vi "Finish.vi"   [LabVIEW 2018]
doc: "This VI is called just before exiting. It is expected to close I/O refnum, save collected data, etc."
uses:
  <vilib>/Rock Robotics/WPI/Utilities/WPI_GetSetVariantRefNum.vi
  <vilib>/Rock Robotics/WPI/Ultrasonic/WPI_SonarSRF04DigitalRefNum Registry Get.vi
  <vilib>/Rock Robotics/WPI/Ultrasonic/WPI_SonarSRF04DigitalClose.vi
types:
  T1 = typedef "WPI_JoystickDevRef.ctl" = cluster{"Device":T2}
  T2 = typedef "WPI_JoystickDeviceEnum.ctl" = enum16{"USB 0", "USB 1", "USB 2", "USB 3", "USB 4", "USB 5"}
  T3 = typedef "WPI_CompressorDevRef.ctl" = cluster{"DevStatus":errorcluster, "Pneumatics Control Module":u8}
  T4 = typedef "WPI_RobotDriveDevRef.ctl" = cluster{"DevStatus":errorcluster, "Motors[]":T5[], "Square Inputs":bool, "Max Output":dbl}
  T5 = typedef "WPI_MotorControlDeviceRef.ctl" = cluster{"DeviceStatus":errorcluster, "Type":T6, "PWM":cluster{"PWM Channel":T7, "DeadBand":T8}, "CAN":cluster{"Device Number":u8, "SetOutput VI Ref":variant, "GetOutput VI Ref":variant, "Enable VI Ref":variant, "Disable VI Ref":variant, "Data":variant}, "Invert":bool, "DIO PWM":cluster{"PWM \"Enable\" Channel":T7, "DIOChannel":T9, "PWM Rate":dbl}}
  T6 = typedef "WPI_MotorControlType.ctl" = enum16{"PWM", "CAN", "DIO PWM"}
  T7 = typedef "FPGA_DIOPWMChannel.ctl" = enum8{"PWM 0", "PWM 1", "PWM 2", "PWM 3", "PWM 4", "PWM 5", "PWM 6", "PWM 7", "PWM 8", "PWM 9", "PWM MXP 0", "PWM MXP 1", "PWM MXP 2", "PWM MXP 3", "PWM MXP 4", "PWM MXP 5", "PWM MXP 6", "PWM MXP 7", "PWM MXP 8", "PWM MXP 9", "Invalid"}
  T8 = typedef "WPI_PWMDeadband.ctl" = cluster{"Name":string, "maxPositivePwm":i32, "minPositivePwm":i32, "centerPwm":i32, "maxNegativePwm":i32, "minNegativePwm":i32, "angularRange":u16}
  T9 = typedef "FPGA_DIOChannel.ctl" = enum8{"DIO 0", "DIO 1", "DIO 2", "DIO 3", "DIO 4", "DIO 5", "DIO 6", "DIO 7", "DIO 8", "DIO 9", "DIO MXP 0", "DIO MXP 1", "DIO MXP 2", "DIO MXP 3", "DIO MXP 4", "DIO MXP 5", "DIO MXP 6", "DIO MXP 7", "DIO MXP 8", "DIO MXP 9", "DIO MXP 10", "DIO MXP 11", "DIO MXP 12", "DIO MXP 13", "DIO MXP 14", "DIO MXP 15", "SPI Port CS1", "SPI Port CS2", "SPI Port CS3", "SPI Port MISO", "SPI Port MOSI", "Invalid"}
  T10 = typedef "WPI_EncoderDevRef.ctl" = cluster{"DevStatus":errorcluster, "EncoderIndex":T11, "CounterIndex":T12, "DistancePerCount":dbl, "Decoding Type":T13}
  T11 = typedef "FPGA_EncoderIdx.ctl" = enum8{"Enc 0", "Enc 1", "Enc 2", "Enc 3", "Enc 4", "Enc 5", "Enc 6", "Enc 7", "Invalid"}
  T12 = typedef "FPGA_CounterCtrSystemIndex.ctl" = enum8{"Ctr 0", "Ctr 1", "Ctr 2", "Ctr 3", "Ctr 4", "Ctr 5", "Ctr 6", "Ctr 7", "Invalid"}
  T13 = typedef "WPI_EncoderType.ctl" = enum16{"1x", "2x", "4x"}
  T14 = typedef "WPI_SwitchDevRef.ctl" = cluster{"DevStatus":errorcluster, "DIO Channel":T9, "CntIndex":T12, "Normally Closed":bool}
  T15 = typedef "WPI_UltrasonicDeviceRef.ctl" = cluster{"DevStatus":errorcluster, "Ping Channel":T9, "Echo Channel":T9, "CntIndex":T12}
  T16 = typedef "WPI_CameraDevRef.ctl" = cluster{"Camera Address":string, "CameraStatus":errorcluster}
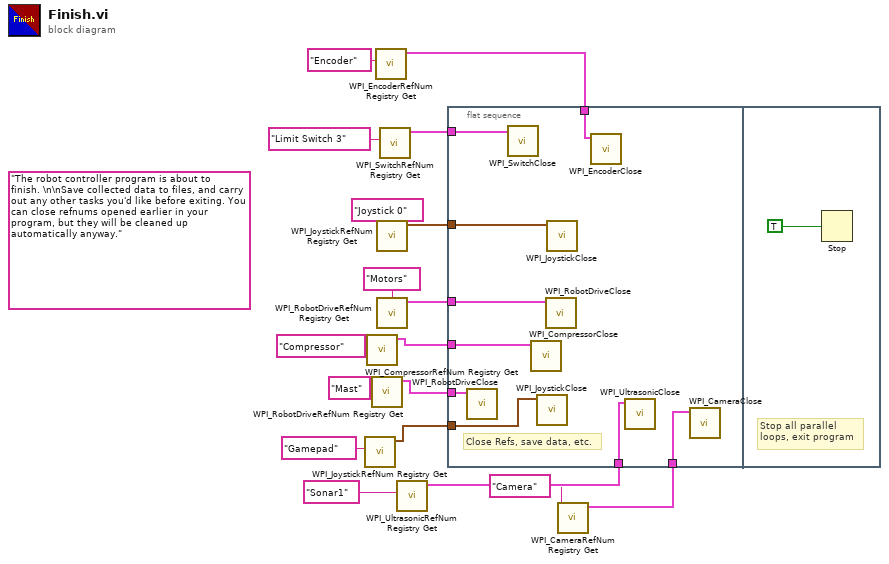
[diagram p0: block diagram]
diagram:
  (unwired) "The robot controller program is about to finish. \n\nSave collected data to files, and carry out any other tasks you'd like before exiting. You can close refnums opened earlier in your program, but they will be cleaned up automatically anyway."
  n1 = call <vilib>:"WPI_JoystickRefNum Registry Get.vi"("refnum name"="Gamepad") -> ("JoystickDevRef"=w12:T1)  [unwired: 1 in, 9 out]
  n2 = call <vilib>:"WPI_CompressorRefNum Registry Get.vi"("refnum name"="Compressor") -> ("CompressorDevRef"=w9:T3)  [unwired: 9 in, 1 out]
  n3 = call <vilib>:"WPI_RobotDriveRefNum Registry Get.vi"("refnum name"="Mast") -> ("RobotDriveDevRef"=w13:T4)  [unwired: 1 in, 9 out]
  n4 = call <vilib>:"WPI_EncoderRefNum Registry Get.vi"("refnum name"="Encoder") -> ("EncoderDevRef"=w2:T10)  [unwired: 9 in, 1 out]
  n5 = call <vilib>:"WPI_JoystickRefNum Registry Get.vi"("refnum name"="Joystick 0") -> ("JoystickDevRef"=w15:T1)  [unwired: 1 in, 9 out]
  n6 = call <vilib>:"WPI_RobotDriveRefNum Registry Get.vi"("refnum name"="Motors") -> ("RobotDriveDevRef"=w16:T4)  [unwired: 1 in, 9 out]
  n7 = call <vilib>:"WPI_SwitchRefNum Registry Get.vi"("refnum name"="Limit Switch 3") -> ("SwitchDevRef"=w4:T14)  [unwired: 9 in, 1 out]
  n8 = call-poly <vilib>:"WPI_UltrasonicRefNum Registry Get.vi"("refnum name"="Sonar1") -> ("SonarSRF04DevRef"=w7:T15)  [unwired: 9 in, 1 out]
  n9 = flat-sequence {
    tunnel: w16 -> [w27]
    tunnel: w15 -> [w26]
    tunnel: w13 -> [w25]
    tunnel: w12 -> [w24]
    tunnel: w9 -> [w23]
    tunnel: w7 -> [w22]
    tunnel: w6 -> [w21]
    tunnel: w4 -> [w20]
    tunnel: w2 -> [w19]
    frame #0 {
      # "Close Refs, save data, etc."
      n10 = call <vilib>:"WPI_RobotDriveClose.vi"("RobotDriveDevRef"=w25) -> ()  [unwired: 1 in, 10 out]
      n11 = call <vilib>:"WPI_SwitchClose.vi"("SwitchDevRef"=w20) -> ()  [unwired: 10 in, 1 out]
      n12 = call <vilib>:"WPI_CompressorClose.vi"("CompressorDevRef"=w23) -> ()  [unwired: 10 in, 1 out]
      n13 = call <vilib>:"WPI_JoystickClose.vi"("JoystickDevRef"=w24) -> ()  [unwired: 11 out]
      n14 = call <vilib>:"WPI_RobotDriveClose.vi"("RobotDriveDevRef"=w27) -> ()  [unwired: 1 in, 10 out]
      n15 = call <vilib>:"WPI_JoystickClose.vi"("JoystickDevRef"=w26) -> ()  [unwired: 11 out]
      n16 = call <vilib>:"WPI_EncoderClose.vi"("EncoderDevRef"=w19) -> ()  [unwired: 10 in, 1 out]
      n17 = call-poly <vilib>:"WPI_UltrasonicClose.vi"("SonarSRF04DevRef"=w22) -> ()  [unwired: 10 in, 1 out]
      n18 = call <vilib>:"WPI_CameraClose.vi"("CameraDevRef"=w21) -> ()  [unwired: 10 in, 1 out]
    }
    frame #1 {
      # "Stop all parallel\nloops, exit program"
      n19 = Stop(stop? (T)=TRUE ("Quit")) -> ()
    }
  }
  n20 = call <vilib>:"WPI_CameraRefNum Registry Get.vi"("refnum name"="Camera") -> ("CameraDevRef"=w6:T16)  [unwired: 9 in, 1 out]
